vi "Read Monitor Data.vi"(8 "error in (no error)":errorcluster, 11 "Actor Monitor New in":refnum<class "Actor Monitor.lvclass">) -> (0 "error out":errorcluster, 2 "Monitored Actor.lvlib:Monitor Data.lvclass":refnum<class "Monitor Data.lvclass">, 3 "Actor Monitor New out":refnum<class "Actor Monitor.lvclass">)   [LabVIEW 2017, in "MGI-Monitored Actor Core.lvlib" / "Actor Monitor.lvclass"]
uses:
  Actor Monitor.lvclass
  Monitor Data/Monitor Data.lvclass
  Actor Monitor.lvclass/Actor Monitor.ctl
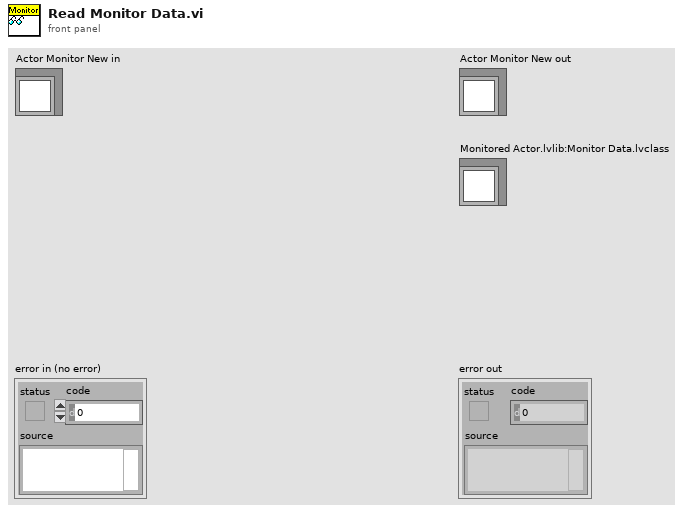
[diagram p1: front panel]
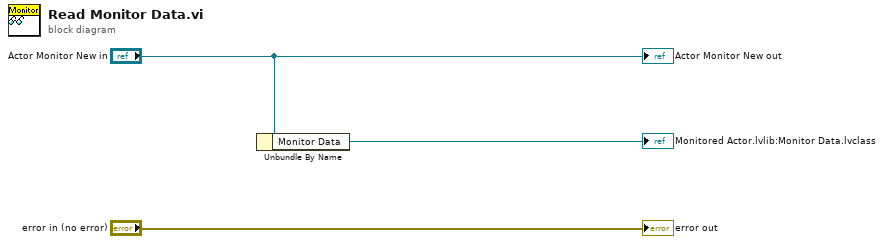
[diagram p0: block diagram]
diagram:
  n1 = Unbundle By Name("Actor Monitor New in") -> ("Monitor Data"=→"Monitored Actor.lvlib:Monitor Data.lvclass":refnum<class "Monitor Data.lvclass">)
  "error out" <- "error in (no error)"
  "Actor Monitor New out" <- "Actor Monitor New in"
